vi "Read Slit Width.vi"(8 "error in (no error)":errorcluster, 11 "VISA resource name":refnum<visa-resource-name>) -> (0 "error out":errorcluster, 2 "Slit Width (um)":i32, 3 "VISA resource name out":refnum<visa-resource-name>, 4 "read buffer":string)   [LabVIEW 2019, in "SpectraPro.lvlib"]
uses:
  SpectraPro.lvlib
panel:
  out "output 2":string
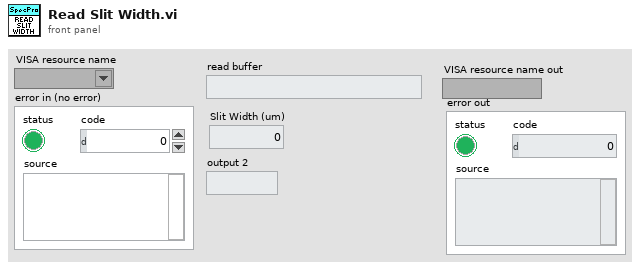
[diagram p1: front panel]
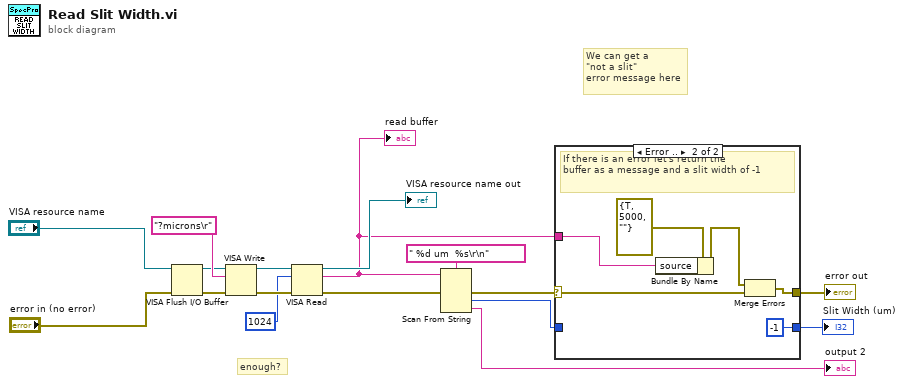
[diagram p0: block diagram]
diagram:
  # "We can get a\n\"not a slit\"\nerror message here"
  # "enough?"
  n1 = VISA Flush I/O Buffer(VISA resource name="VISA resource name", error in (no error)="error in (no error)") -> (VISA resource name out=w1:refnum<visa-resource-name>, error out=w3:errorcluster)  [unwired: 1 in]
  n2 = VISA Write(VISA resource name=w1, write buffer="?microns\r", error in (no error)=w3) -> (VISA resource name out=w15:refnum<visa-resource-name>, error out=w16:errorcluster)  [unwired: 1 out]
  n3 = VISA Read(VISA resource name=w15, byte count=u32 1024, error in (no error)=w16) -> (VISA resource name out=→"VISA resource name out":refnum<visa-resource-name>, read buffer=w4:string, error out=w9:errorcluster)  [unwired: 1 out]
  "read buffer" <- w4
  n4 = Scan From String(format string=" %d um  %s\r\n", input string=w4, error in=w9) -> (error out=w8:errorcluster, output 1=w5:i32, output 2=→"output 2":string)  [unwired: 3 in, 2 out]
  n5 = case shown="Error .." w8 {
    selector: w8 -> [w19 w25]
    tunnel: [w19 w24] -> w7
    tunnel: [w18 -1] -> w6
    tunnel: w5 -> [w18 _]
    tunnel: w4 -> [_ w21]
    frame No Error {
    }
    frame Error {
      # "If there is an error let's return the\nbuffer as a message and a slit width of -1"
      n6 = Bundle By Name(cluster=errorcluster {"status"=TRUE, "code"=5000, "source"=""} ("error in (no error)"), "source"=w21) -> (w22:errorcluster)
      n7 = Merge Errors(w22, w25) -> (w24:errorcluster)
    }
  }
  "error out" <- w7
  "Slit Width (um)" <- w6
